vi "Neocera21 Get T - V1.vi"(8 "error in (no error)":errorcluster, 10 "Sensor":i32=1, 11 "VISA Resource Name":refnum<visa-resource-name>) -> (0 "error out":errorcluster, 1 "data string":string, 2 "Temperature":dbl format="%.2f", 3 "VISA Resource Name Out":refnum<visa-resource-name>)   [LabVIEW 2014]
uses:
  GPIB.llb/VISA  Send Receive.vi
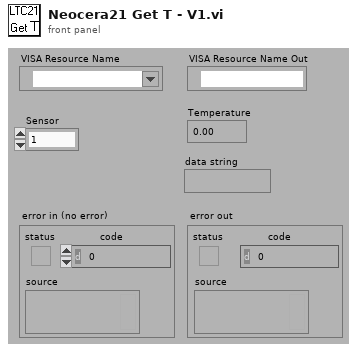
[diagram p1: front panel]
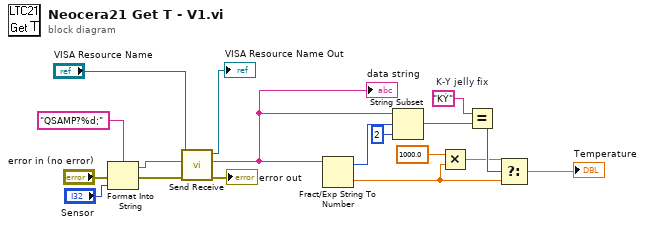
[diagram p0: block diagram]
diagram:
  w7 = "KÝ"  # K-Y jelly fix
  n1 = Format Into String(format string="QSAMP?%d;" ("data string"), error in="error in (no error)", "Sensor") -> (resulting string=w11:string, error out=w12:errorcluster)  [unwired: 1 in]
  n2 = call-poly "Send Receive.vi"("error in (no error)"=w12, "data string in"=w11, "VISA Resource Name"="VISA Resource Name") -> ("error out"=→"error out":errorcluster, "data string out"=w10:string, "VISA Resource Name Out"=→"VISA Resource Name Out":refnum<visa-resource-name>)  [unwired: 6 in]
  "data string" <- w10
  n3 = Fract/Exp String To Number(string=w10) -> (offset past number=w9:i32, number=w3:dbl)  [unwired: 3 out]
  n4 = String Subset(string=w10, offset (0)=w9, length (rest)=2 ("length (rest)")) -> (substring=w6:string)
  n5 = Multiply(x=1000.0, y=w3) -> (x*y=w1:dbl)
  n6 = Equal?(x=w7, y=w6) -> (x = y?=w5:bool)
  n7 = Select(t=w1, s=w5, f=w3) -> (s? t:f=→"Temperature":dbl)
